vi "Simulator Play Sound.vi"(8 "error in (no error)":errorcluster, 11 "Sound File Path":string) -> (0 "error out":errorcluster)   [LabVIEW 2014]
doc: "This VI illustrates how to play a sound file continuously, reading the sound file in pieces, and playing each piece at a time."
uses:
  <vilib>/sound2/lvsound2.llb/Sampling Mode.ctl
  <vilib>/sound2/lvsound2.llb/Sound File Info (path).vi
  <vilib>/sound2/lvsound2.llb/Sound File Read Open.vi
  <vilib>/sound2/lvsound2.llb/Sound File Read (DBL).vi
  <vilib>/sound2/lvsound2.llb/Sound Output Write (DBL).vi
panel:
  in  "Device ID":u32
  # "Overview: Demonstrates the use of the Sound VIs to play a sound file continuously, reading the sound file in pieces, and playing each piece one at a time.\nInstructions:\n1. Specify the Device ID and the Number of Samples/Iteration.\n2. Run the VI."
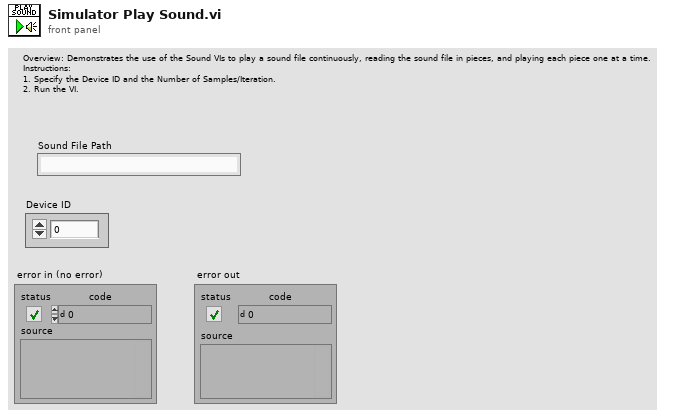
[diagram p1: front panel]
types:
  T1 = typedef "Sampling Mode.ctl" = i32
  T2 = typedef "Sound Data Format.ctl" = cluster{"sample rate (S/s)":dbl, "number of channels":i32, "bits per sample":i32}
  T3 = typedef "Sound File Refnum.ctl" = refnum<file>
  T4 = typedef "Sound Output Task ID.ctl" = u32
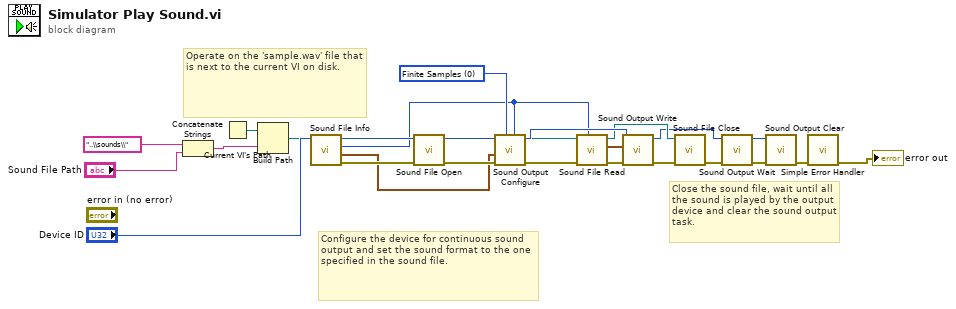
[diagram p0: block diagram]
diagram:
  w11 = T1 0 items=["Finite Samples", "Continuous Samples"] ("sample mode")
  # "Operate on the 'sample.wav' file that is next to the current VI on disk."
  # "Close the sound file, wait until all the sound is played by the output device and clear the sound output task."
  # "Configure the device for continuous sound output and set the sound format to the one specified in the sound file."
  n1 = Concatenate Strings("..\\sounds\\" ("string"), "Sound File Path") -> (w7:string)
  n2 = Current VI's Path() -> (path=w8:path)
  n3 = Build Path(base path=w8, name or relative path=w7) -> (appended path=w9:path)
  n4 = call-poly <vilib>:"Sound File Info.vi"("path"=w9) -> ("error out"=w20:errorcluster, "sound format"=w12:T2, "total number of samples/ch"=w4:u32, "path out"=w13:path)  [unwired: 7 in]
  n5 = call-poly <vilib>:"Sound File Open.vi"("error in (no error)"=w20, "path"=w13) -> ("error out"=w19:errorcluster, "sound file refnum"=w21:T3)  [unwired: 8 in]
  n6 = call <vilib>:"Sound Output Configure.vi"("number of samples/ch"=w4, "sample mode"=w11, "error in (no error)"=w19, "sound format"=w12, "device ID"="Device ID") -> ("error out"=w18:errorcluster, "task ID"=w25:T4)  [unwired: 5 in]
  n7 = call-poly <vilib>:"Sound File Read.vi"("number of samples/ch (-1: all)"=w4, "error in (no error)"=w18, "sound file refnum"=w21) -> ("error out"=w3:errorcluster, "data"=w2:waveform(dbl)[], "sound file refnum out"=w23:T3)  [unwired: 4 in, 2 out]
  n8 = call-poly <vilib>:"Sound Output Write.vi"("error in (no error)"=w3, "data"=w2, "task ID"=w25) -> ("error out"=w22:errorcluster, "task ID out"=w16:T4)  [unwired: 7 in]
  n9 = call <vilib>:"Sound File Close.vi"("error in (no error)"=w22, "sound file refnum"=w23) -> ("error out"=w15:errorcluster)  [unwired: 9 in]
  n10 = call <vilib>:"Sound Output Wait.vi"("error in (no error)"=w15, "task ID"=w16) -> ("error out"=w14:errorcluster, "task ID out"=w17:T4)  [unwired: 8 in]
  n11 = call <vilib>:"Sound Output Clear.vi"("error in (no error)"=w14, "task ID"=w17) -> ("error out"=w10:errorcluster)  [unwired: 9 in]
  n12 = call <vilib>:"Simple Error Handler.vi"("error in (no error)"=w10) -> ("error out"=→"error out":errorcluster)  [unwired: 4 in, 4 out]
